vi "Implode String.vi"(7 "Delimiter (comma)":string=",", 11 "String Array":string[](array[string])) -> (3 "Imploded String":string)   [LabVIEW 2018, in "IO.lvlib"]
uses:
  IO.lvlib
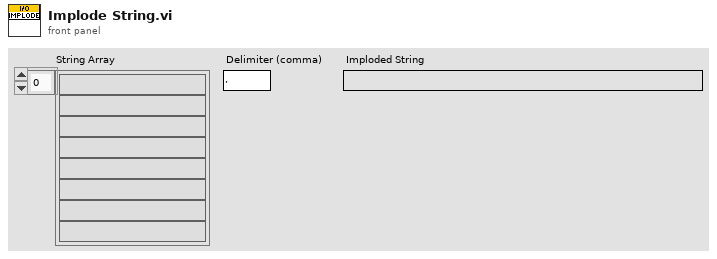
[diagram p1: front panel]
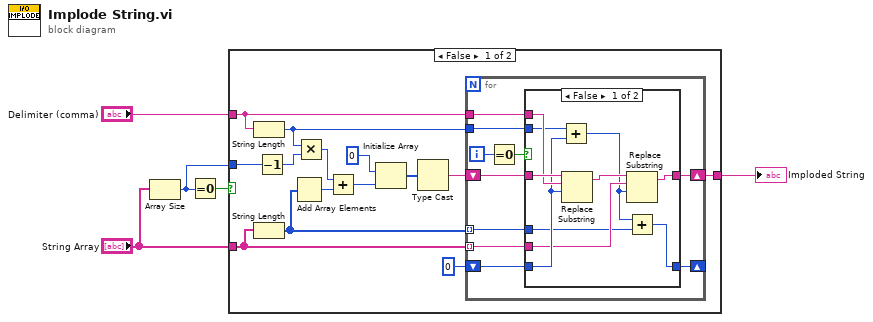
[diagram p0: block diagram]
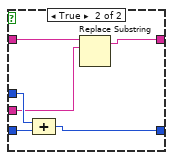
[diagram p2: hidden frame]
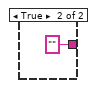
[diagram p3: hidden frame]
diagram:
  n1 = Array Size(array="String Array") -> (size(s)=w4:i32)
  n2 = Equal To 0?(x=w4) -> (x = 0?=w3:bool)
  n3 = case shown="False" w3 {
    tunnel: "Delimiter (comma)" -> [w9 _]
    tunnel: w4 -> [w18 _]
    tunnel: "String Array" -> [w10 _]
    tunnel: [w6 ""] -> w1
    frame False {
      n4 = String Length(string=w9) -> (length=w7:i32)
      n5 = String Length(string=w10) -> (length=w8:i32[])
      n6 = Decrement(x=w18) -> (x-1=w19:i32)
      n7 = Add Array Elements(numeric array=w8) -> (sum=w17:i32)
      n8 = Multiply(x=w7, y=w19) -> (x*y=w16:i32)
      n9 = Add(x=w16, y=w17) -> (x+y=w15:i32)
      n10 = Initialize Array(u8 0 ("element"), w15) -> (w13:u8[])
      n11 = Type Cast(x=w13) -> (*(type *) &x=w11:string)  [unwired: 1 in]
      n12 = for {
        shift-right: [w21] -> _
        shift-left: 0 -> [w23]
        shift-right: [w20] -> w6
        shift-left: w11 -> [w25]
        tunnel: w10 -> [w28] mode=indexing
        tunnel: w9 -> [w26]
        tunnel: w8 -> [w24] mode=indexing
        tunnel: w7 -> [w22]
        i -> [w29]
        n13 = Equal To 0?(x=w29) -> (x = 0?=w27:bool)
        n14 = case shown="False" w27 {
          tunnel: w28 -> [w35 w41]
          tunnel: w26 -> [w38 _]
          tunnel: w25 -> [w39 w42]
          tunnel: w24 -> [w32 w44]
          tunnel: w23 -> [w36 w45]
          tunnel: w22 -> [w37 _]
          tunnel: [w30 w43] -> w21
          tunnel: [w33 w40] -> w20
          frame False {
            n15 = Add(x=w37, y=w36) -> (x+y=w31:i32)
            n16 = Replace Substring(3:w36, 4:w38, 5:w39) -> (1:w34:string)  [unwired: 1 in, 1 out]
            n17 = Replace Substring(3:w31, 4:w35, 5:w34) -> (1:w33:string)  [unwired: 1 in, 1 out]
            n18 = Add(x=w31, y=w32) -> (x+y=w30:i32)
          }
          frame True {
            n19 = Compound Arithmetic op=ADD(w44, w45) -> (w43:i32)
            n20 = Replace Substring(4:w41, 5:w42) -> (1:w40:string)  [unwired: 2 in, 1 out]
          }
        }
      }
    }
    frame True {
    }
  }
  "Imploded String" <- w1
